vi "Reset.vi"(8 "error in (no error)":errorcluster, 11 "Process Tree View in":refnum<class "Process Tree View.lvclass">) -> (0 "error out":errorcluster, 3 "Process Tree View out":refnum<class "Process Tree View.lvclass">)   [LabVIEW 2020, in "Process Tree View.lvclass"]
uses:
  Process Tree View.lvclass
  Process Tree View.lvclass/Process Tree View.ctl
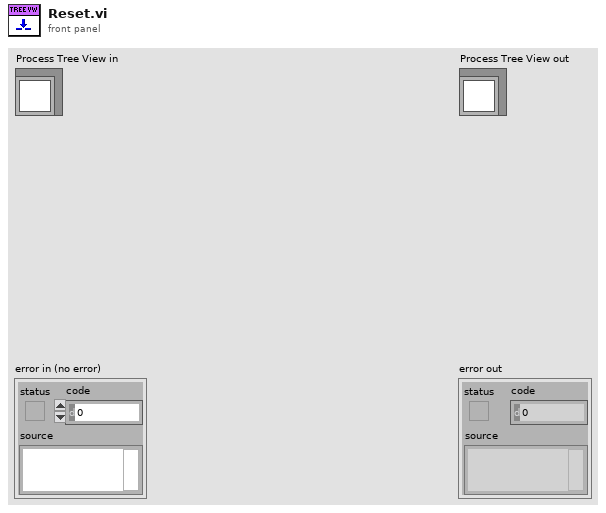
[diagram p1: front panel]
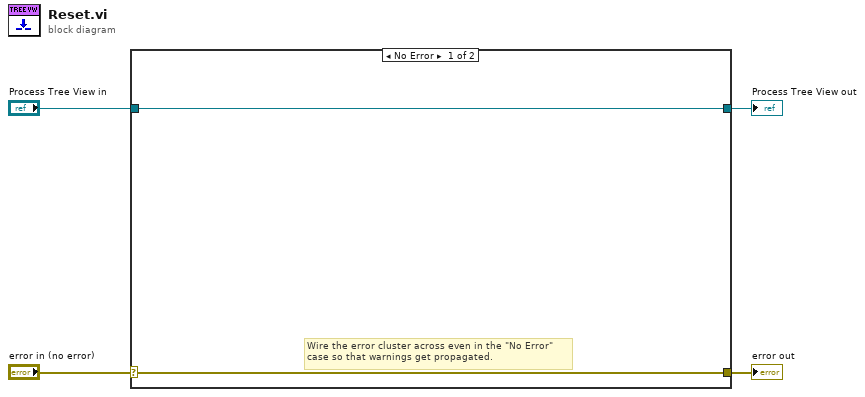
[diagram p0: block diagram]
diagram:
  n1 = case shown="No Error" "error in (no error)" {
    selector: "error in (no error)" -> [w5 w8]
    tunnel: [w5 w8] -> w3
    tunnel: [w6 w7] -> w1
    tunnel: "Process Tree View in" -> [w6 w7]
    frame No Error {
      # "Wire the error cluster across even in the \"No Error\"\ncase so that warnings get propagated."
    }
    frame Error {
    }
  }
  "error out" <- w3
  "Process Tree View out" <- w1
